vi "GetLastEvent.vi"(7 "LabVIEW Web Service Request":refnum<class "Web Request.lvclass">, 11 "Asset":string) -> (3 "Output":T2(array[cluster]))   [LabVIEW 2017]
uses:
  <vilib>/wsapi/Web Request.lvclass
  <vilib>/addons/InsightCM/MessageBus/Base/controls/KeyValuePair.ctl
panel:
  # "Use the Web Service Request input terminal to call the VIs on the Web Services palette. Do not remove it from the connector pane unless you don't need access to the palette."
  # "Each additional control wired to the connector pane will be available as an input in the URL. To include an indicator in terminal-mode output (the default setting), it must also be wired to the connector pane."
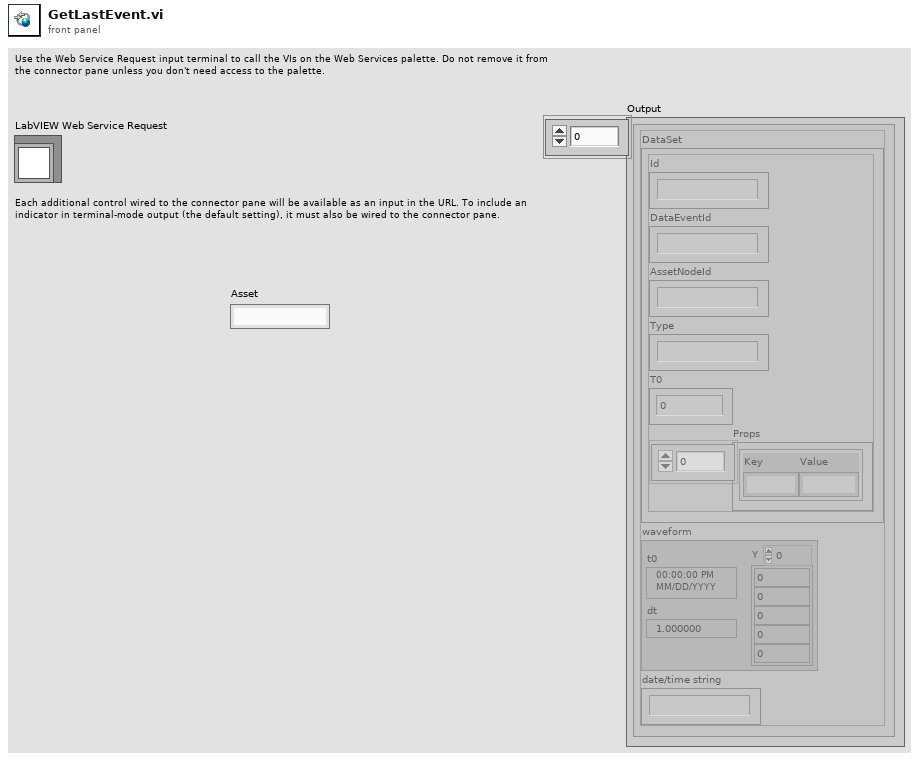
[diagram p1: front panel]
types:
  T1 = typedef "KeyValuePair.ctl" = cluster{"Key":string, "Value":string}
  T2 = cluster{"DataSet":cluster{"Id":string, "DataEventId":string, "AssetNodeId":string, "Type":string, "T0":i64, "Props":T1[]}, "waveform":waveform(sgl), "date/time string":string}[]
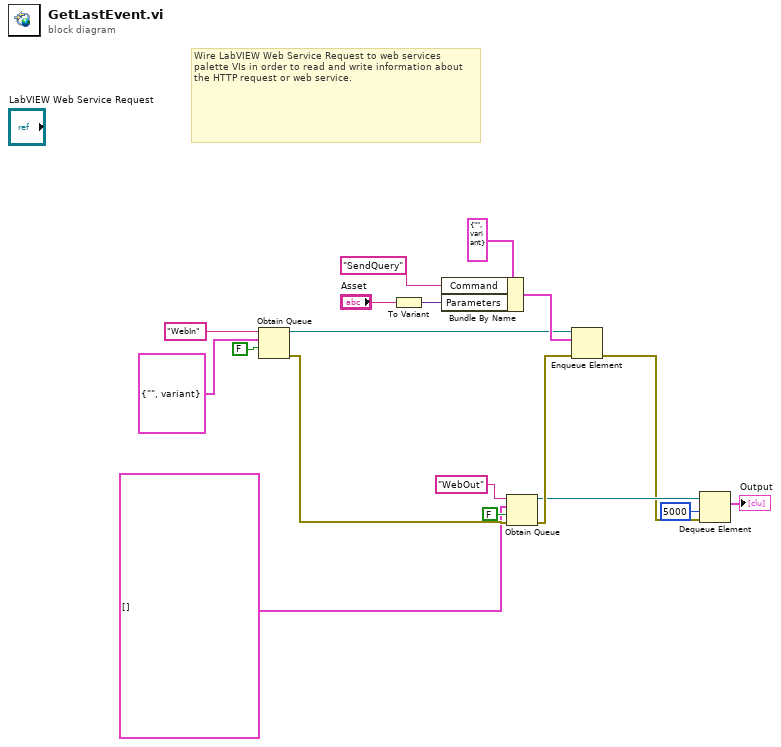
[diagram p0: block diagram]
diagram:
  # "Wire LabVIEW Web Service Request to web services palette VIs in order to read and write information about the HTTP request or web service."
  n1 = Obtain Queue(name (unnamed)="WebIn", element data type=cluster{"Command":string, "Parameters":variant} {"Command"="", "Parameters"=variant}, create if not found? (T)=FALSE) -> (queue out=w11:refnum<queue>, error out=w8:errorcluster)  [unwired: 2 in, 1 out]
  n2 = To Variant(anything="Asset") -> (Variant=w14:variant)
  n3 = Bundle By Name(cluster=cluster{"Command":string, "Parameters":variant} {"Command"="", "Parameters"=variant} ("element"), "Command"="SendQuery", "Parameters"=w14) -> (w13:cluster{"Command":string, "Parameters":variant})
  n4 = Obtain Queue(name (unnamed)="WebOut", element data type=T2 [] ("Output"), create if not found? (T)=FALSE, error in (no error)=w8) -> (queue out=w5:refnum<queue>, error out=w6:errorcluster)  [unwired: 1 in, 1 out]
  n5 = Enqueue Element(queue=w11, element=w13, error in (no error)=w6) -> (error out=w4:errorcluster)  [unwired: 1 in, 2 out]
  n6 = Dequeue Element(queue=w5, timeout in ms (-1)=5000, error in (no error)=w4) -> (element=→"Output":T2)  [unwired: 3 out]
